vi "Clear All Children.vi"(8 "error in (no error)":errorcluster, 11 "Item Ref in":T1 format="%.0x") -> (0 "error out":errorcluster, 3 "Section Ref out":T1 format="%.0x")   [LabVIEW 2015, in "NI 9759 RevB Custom Device.lvlib"]
uses:
  <vilib>/NI Veristand/Custom Device API/Custom Device Item Ref.ctl
  NI 9759 RevB Custom Device.lvlib
  <vilib>/NI VeriStand/Custom Device API/Custom Device API.lvlib
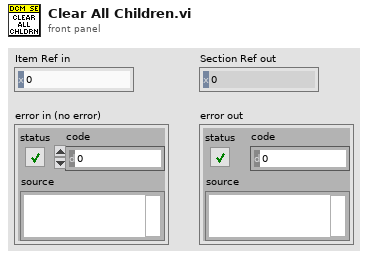
[diagram p1: front panel]
types:
  T1 = typedef "Custom Device API.lvlib/Custom Device Item Ref.ctl" = u64
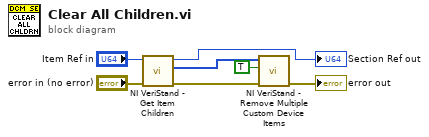
[diagram p0: block diagram]
diagram:
  n1 = call <vilib>:"NI VeriStand - Get Item Children.vi"("error in (no error)"="error in (no error)", "Item Ref in"="Item Ref in") -> ("error out"=w4:errorcluster, "Child Refs"=w2:T1[], "Item Ref out"=→"Section Ref out":T1)  [unwired: 6 in, 1 out]
  n2 = call <vilib>:"NI VeriStand - Remove Multiple Custom Device Items.vi"("error in (no error)"=w4, "Force Delete (F)"=TRUE, "Item Refs in"=w2) -> ("error out"=→"error out":errorcluster)  [unwired: 7 in, 1 out]
